vi "Boatloader_Msg_Entry_Exit.vi"(0 "Frame":string, 5 "dst":string, 7 "CMD":string, 9 "Msg":string) -> (8 "Message":string)   [LabVIEW 2021]
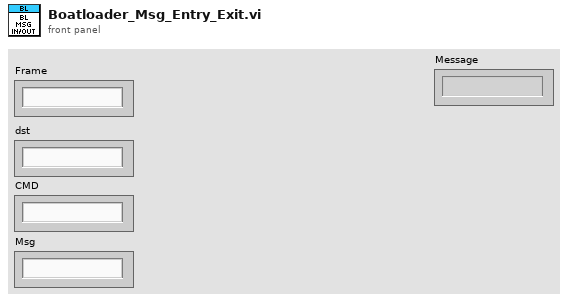
[diagram p1: front panel]
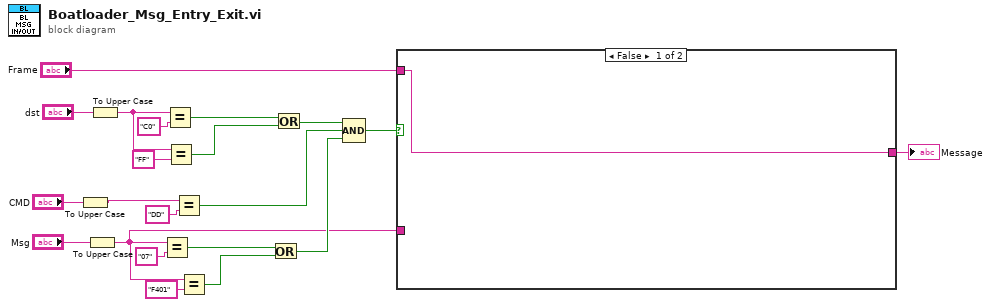
[diagram p0: block diagram]
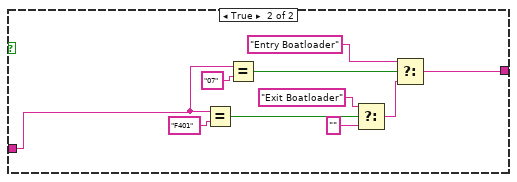
[diagram p2: hidden frame]
diagram:
  n1 = To Upper Case(1:"CMD") -> (0:w13:string)
  n2 = To Upper Case(1:"Msg") -> (0:w2:string)
  n3 = To Upper Case(1:"dst") -> (0:w17:string)
  n4 = Equal?(x=w2, y="07") -> (x = y?=w9:bool)
  n5 = Equal?(x=w17, y="C0") -> (x = y?=w18:bool)
  n6 = Equal?(x=w17, y="FF") -> (x = y?=w15:bool)
  n7 = Equal?(x=w13, y="DD") -> (x = y?=w5:bool)
  n8 = Equal?(x=w2, y="F401") -> (x = y?=w11:bool)
  n9 = Or(x=w9, y=w11) -> (x .or. y?=w3:bool)
  n10 = Or(x=w18, y=w15) -> (x .or. y?=w6:bool)
  n11 = Compound Arithmetic op=AND(w6, w5, w3) -> (w4:bool)
  n12 = case shown="False" w4 {
    tunnel: [w22 w24] -> w12
    tunnel: w2 -> [_ w23]
    tunnel: "Frame" -> [w22 _]
    frame False {
    }
    frame True {
      n13 = Equal?(x=w23, y="F401") -> (x = y?=w32:bool)
      n14 = Equal?(x=w23, y="07") -> (x = y?=w30:bool)
      n15 = Select(t="Exit Boatloader" ("y"), s=w32, f="") -> (s? t:f=w31:string)
      n16 = Select(t="Entry Boatloader" ("y"), s=w30, f=w31) -> (s? t:f=w24:string)
    }
  }
  "Message" <- w12
